vi "Configure Waveform Shape.vi"(7 "Select Output Waveform (0:Waveform A)":u16(ring) items=["Waveform A", "Waveform B"], 8 "error in (no error)":errorcluster, 9 "Wave Variable (0)":u32 max=100, 10 "Waveform (0:Sine)":u16(ring) items=["Sine", "Square", "Clipped", "THD", "User"], 11 "VISA resource name":refnum<visa-resource-name>) -> (0 "error out":errorcluster, 3 "VISA resource name out":refnum<visa-resource-name>)   [LabVIEW 2015, in "BK Precision 983X Series.lvlib"]
doc: "Selects and configures the waveform shape to use for the AC output."
uses:
  <instrlib>/BK Precision 983X Series/BK Precision 983X Series.lvlib
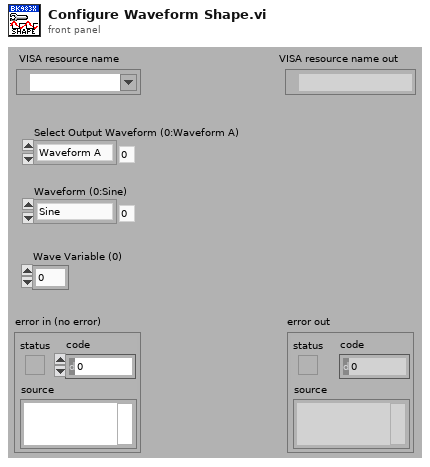
[diagram p1: front panel]
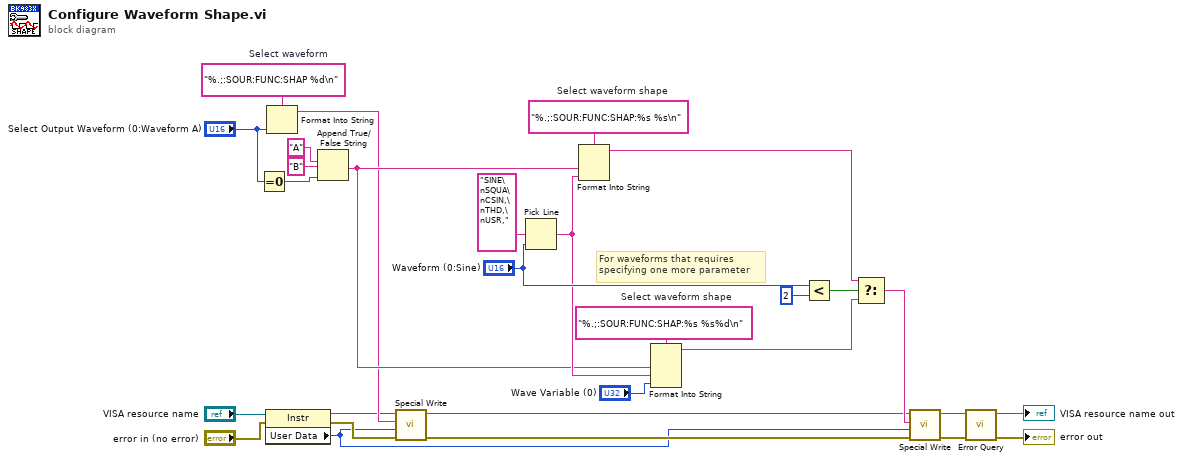
[diagram p0: block diagram]
diagram:
  w12 = "%.;:SOUR:FUNC:SHAP:%s %s%d\n"  # Select waveform shape
  w22 = "%.;:SOUR:FUNC:SHAP %d\n"  # Select waveform
  w27 = "%.;:SOUR:FUNC:SHAP:%s %s\n"  # Select waveform shape
  # "For waveforms that requires\nspecifying one more parameter"
  n1 = Equal To 0?(x="Select Output Waveform (0:Waveform A)") -> (x = 0?=w19:bool)
  n2 = property class="Instr"(reference="VISA resource name", error in="error in (no error)") -> (reference out=w5:refnum<visa-resource-name>, error out=w4:errorcluster, "User Data"=w1:u32)
  n3 = Format Into String(format string=w22, "Select Output Waveform (0:Waveform A)") -> (resulting string=w6:string)  [unwired: 2 in, 1 out]
  n4 = Append True/False String(1:w19, 2:"B" ("false string"), 3:"A" ("true string")) -> (0:w9:string)  [unwired: 1 in]
  n5 = call <instrlib>:"Special Write.vi"("error in (no error)"=w4, "Delay (0 ms)"=w1, "Input String"=w6, "VISA resource name"=w5) -> ("error out"=w2:errorcluster, "VISA resource name out"=w3:refnum<visa-resource-name>)  [unwired: 6 in]
  n6 = Pick Line(multi-line string="SINE\nSQUA\nCSIN,\nTHD,\nUSR,", line index="Waveform (0:Sine)") -> (output string=w10:string)  [unwired: 1 in]
  n7 = Format Into String(format string=w27, w9, w10) -> (resulting string=w13:string)  [unwired: 2 in, 1 out]
  n8 = Format Into String(format string=w12, w9, w10, "Wave Variable (0)") -> (resulting string=w8:string)  [unwired: 2 in, 1 out]
  n9 = Less?(x="Waveform (0:Sine)", y=u16 2) -> (x < y?=w14:bool)
  n10 = Select(t=w13, s=w14, f=w8) -> (s? t:f=w7:string)
  n11 = call <instrlib>:"Special Write.vi"("error in (no error)"=w2, "Delay (0 ms)"=w1, "Input String"=w7, "VISA resource name"=w3) -> ("error out"=w23:errorcluster, "VISA resource name out"=w24:refnum<visa-resource-name>)  [unwired: 6 in]
  n12 = call <instrlib>:"Error Query.vi"("error in (no error)"=w23, "VISA resource name"=w24) -> ("error out"=→"error out":errorcluster, "VISA resource name out"=→"VISA resource name out":refnum<visa-resource-name>)  [unwired: 6 in, 2 out]
